vi "GenNet Format System Message for MsgQ.vi"(9 "Payload":variant, 10 "Sys. Msg. Origin":string, 11 "Identifer":string) -> (2 "System Message Argument":T1, 3 "System Message constant":string)   [LabVIEW 2020, in "hse-gennet.lvlib"]
doc: "Formats the contents of a System Message\n\n____\nHAMPEL SOFTWARE ENGINEERING v3.8.0 (2023-12-18 14:41)"
uses:
  hse-gennet.lvlib
  hse-dqmh/Controls/System Message Argument--cluster.ctl
  hse-dqmh/Controls/System Message Source.ctl
  hse-dqmh/hse-dqmh.lvlib
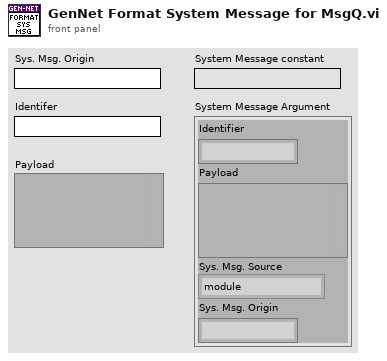
[diagram p1: front panel]
types:
  T1 = typedef "hse-dqmh.lvlib/System Message Argument--cluster.ctl" = cluster{"Identifier":string, "Payload":variant, "Sys. Msg. Source":T2, "Sys. Msg. Origin":string}
  T2 = typedef "hse-dqmh.lvlib/System Message Source.ctl" = enum16{"module", "application", "network"}
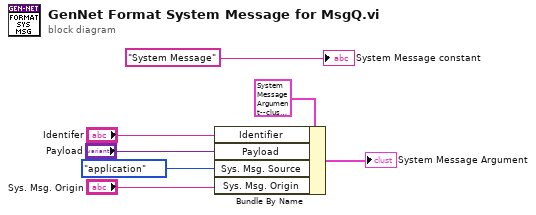
[diagram p0: block diagram]
diagram:
  n1 = Bundle By Name(cluster=T1 {"Identifier"="", "Payload"=variant, "Sys. Msg. Source"=enum."module", "Sys. Msg. Origin"=""} ("System Message Argument"), "Identifier"="Identifer", "Payload"="Payload", "Sys. Msg. Source"=System_Message_Source."application" ("System Message Source"), "Sys. Msg. Origin"="Sys. Msg. Origin") -> (→"System Message Argument":T1)
  "System Message constant" <- "System Message" ("Message")
